vi "ROI group-Set ROIs visibility.vi"(8 "error in (no error)":errorcluster, 9 "Visible?":bool=TRUE, 11 "Indexes of new ROIs to make visible":i32[](array[numeric])) -> (0 "error out":errorcluster)   [LabVIEW 2020]
uses:
  Global variables/gl_Functional Imaging-Global variables.vi
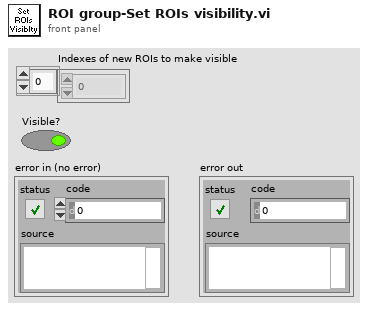
[diagram p1: front panel]
types:
  T1 = typedef "Functional Imging UI Refs.ctl" = cluster{"Menu ref":refnum<k9>, "Image control":refnum<vi>, "VI ref":refnum<vi>, "XGrapher":refnum<vi>, "Smoothing":refnum<vi>, "POI Averaging":refnum<vi>, "Normalize":refnum<vi>, "POI data points in each trial":refnum<vi>, "Channel":refnum<vi>, "Experiment data folder path":refnum<vi>, "[ROI vis]":refnum<vi>, "[Groups] visbl":T2, "Group Name":refnum<vi>, "POI index":refnum<vi>, "Trial No.":refnum<vi>, "Intensity Zoom":refnum<vi>, "Trial Cursor Enabled":refnum<vi>, "Number of Trials (ind 1)":refnum<vi>, "Number of Trials (ind 2)":refnum<vi>, "MiniScans Available":refnum<vi>, "POI Available":refnum<vi>, "Defer graph updates":refnum<vi>, "Waveform selector":refnum<vi>, "#of selected POI":refnum<vi>, "#of selected MiniScans":refnum<vi>, "#of selected groups":refnum<vi>, "Max Z-Projection":refnum<vi>, "Z-Plane Selector":refnum<vi>, "Index of miniscan point to visualise":refnum<vi>, "ROI vis. mode":refnum<vi>, "Total # of points":refnum<vi>, "Index of group clicked on":refnum<vi>, "Pane 1":refnum<vi>, "Pane 2":refnum<vi>, "Pane 3":refnum<vi>, "Pane 4":refnum<vi>, "Pane 5":refnum<vi>, "Pane 6":refnum<vi>, "Deselect all ROI":refnum<vi>, "Deselect all groups":refnum<vi>}
  T2 = typedef "Groups array referecne.ctl" = refnum<vi>
  T3 = typedef "ROI selector array-ROI vis.ctl" = T4[]
  T4 = typedef "Interface-ROI selection cluster.ctl" = cluster{"ROI number":i32, "ROI ID":T5, "Visibility":bool}
  T5 = typedef "ROI ID Enum.ctl" = enum16{"Point", "MiniScan", "Comp. MiniScan", "Rectangle", "Comp. volume", "Arb. plane point", "None"}
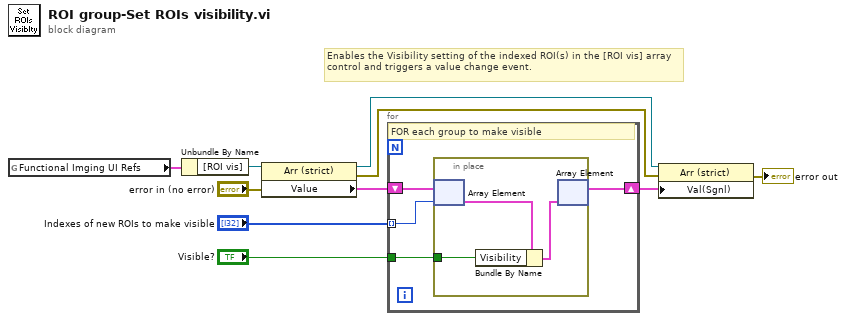
[diagram p0: block diagram]
diagram:
  # "Enables the Visibility setting of the indexed ROI(s) in the [ROI vis] array control and triggers a value change event."
  n1 = global read "gl_Functional Imaging-Global variables.vi" "Functional Imging UI Refs"() -> (w4:T1)
  n2 = Unbundle By Name(w4) -> ("[ROI vis]"=w5:refnum<vi>)
  n3 = property on="Property Node" class="Arr (strict)"(reference=w5, error in="error in (no error)") -> (reference out=w6:refnum<vi>, error out=w8:errorcluster, "Value"=w7:T3)
  n4 = for {
    shift-right: [w13] -> w3
    shift-left: w7 -> [w14]
    tunnel: "Indexes of new ROIs to make visible" -> [w12] mode=indexing
    tunnel: "Visible?" -> [w11]
    # "FOR each group to make visible"
    n5 = in-place "In Place Element Structure" {
      in-place-border: w11 -> [w15]
      n6 = in-place-array #1(w14, w12) -> (w17:T4)
      n7 = Bundle By Name(cluster=w17, "Visibility"=w15) -> (w16:T4)
      n8 = in-place-array #1(w16) -> (w13:T3)  [unwired: 1 out]
    }
  }
  n9 = property on="Property Node" class="Arr (strict)"(reference=w6, error in=w8, "Val(Sgnl)"=w3) -> (error out=→"error out":errorcluster)  [unwired: 1 out]
